vi "Trigger Detector.vi"   [LabVIEW 2014, in "NI_EP_Power Quality.lvlib"]
doc: "Detects crossing of limits for the measurement that you specify and returns triggers if occur.\n\nThis VI supports measuring single-line and multiple-line systems except the DBL instance. Use the DBL instance to measure one channel on one line at one time."
uses:
  <vilib>/addons/Electrical Power/PQ/NI_EP_Power Quality.lvlib
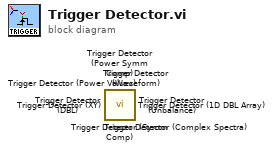
[diagram p0: block diagram]
diagram:
  n1 = call <vilib>:"Trigger Detector (Symm Comp).vi"() -> ()  [unwired: 13 in, 3 out]
  n2 = call <vilib>:"Trigger Detector (Waveform).vi"() -> ()  [unwired: 13 in, 3 out]
  n3 = call <vilib>:"Trigger Detector (XY).vi"() -> ()  [unwired: 13 in, 3 out]
  n4 = call <vilib>:"Trigger Detector (Unbalance).vi"() -> ()  [unwired: 13 in, 3 out]
  n5 = call <vilib>:"Trigger Detector (Power Values).vi"() -> ()  [unwired: 13 in, 3 out]
  n6 = call <vilib>:"Trigger Detector (Power Symm Comp).vi"() -> ()  [unwired: 13 in, 3 out]
  n7 = call <vilib>:"Trigger Detector (Complex Spectra).vi"() -> ()  [unwired: 13 in, 3 out]
  n8 = call <vilib>:"Trigger Detector (1D DBL Array).vi"() -> ()  [unwired: 13 in, 3 out]
  n9 = call <vilib>:"Trigger Detector (DBL).vi"() -> ()  [unwired: 13 in, 3 out]
